vi "createEventForceActuatorInfo.vi"(8 "error in (no error)":errorcluster, 11 "UserEvents in":refnum<class "UserEvents.lvclass">) -> (0 "error out":errorcluster, 3 "UserEvents out":refnum<class "UserEvents.lvclass">)   [LabVIEW 2016, in "UserEvents.lvclass"]
uses:
  UserEvents.lvclass
  DataTypes/Topics/EventForceActuatorInfo.ctl
  DataTypes/Topics/Parts/Timestamp.ctl
  UserEvents.lvclass/UserEvents.ctl
  DataTypes/Topics/M1M3SupportTopics.lvlib
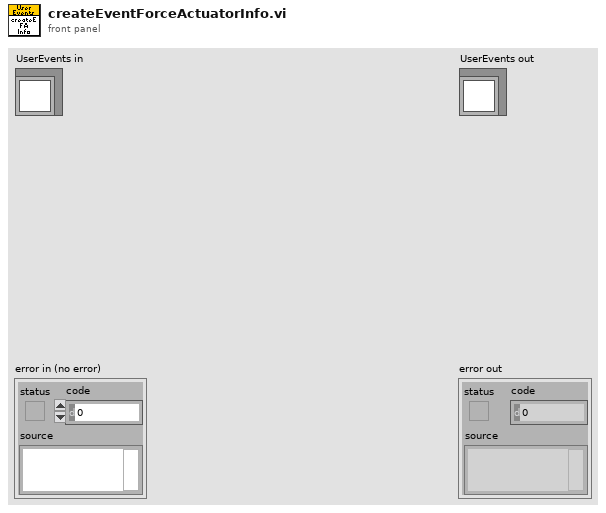
[diagram p1: front panel]
types:
  T1 = typedef "M1M3SupportTopics.lvlib/EventForceActuatorInfo.ctl" = cluster{"Timestamp":T2, "ReferenceId":i32[], "XPosition":sgl[], "YPosition":sgl[], "ZPosition":sgl[], "ILCUniqueId":i64[], "ILCApplicationType":u8[], "NetworkNodeType":u8[], "ILCSelectedOptions":u8[], "NetworkNodeOptions":u8[], "MajorRevision":u8[], "MinorRevision":u8[], "ADCScanRate":u8[], "MainADCCalibrationK1":sgl[], "MainADCCalibrationK2":sgl[], "MainADCCalibrationK3":sgl[], "MainADCCalibrationK4":sgl[], "MainAxialLoadCellOffset":sgl[], "MainLateralLoadCellOffset":sgl[], "MainAxialLoadCellSensitivity":sgl[], "MainLateralLoadCellSensitivity":sgl[], "BackupADCCalibrationK1":sgl[], "BackupADCCalibrationK2":sgl[], "BackupADCCalibrationK3":sgl[], "BackupADCCalibrationK4":sgl[], "BackupAxialLoadCellOffset":sgl[], "BackupLateralLoadCellOffset":sgl[], "BackupAxialLoadCellSensitivity":sgl[], "BackupLateralLoadCellSensitivity":sgl[], "DCAAxialGain":sgl[], "DCALateralGain":sgl[], "DCAUniqueId":i64[], "DCAFirmwareType":u8[], "DCAMajorRevision":u8[], "DCAMinorRevision":u8[], "MainCalibrationError":bool[], "BackupCalibrationError":bool[], "DCAFirmwareUpdate":bool[], "UniqueIdCRCError":bool[], "ApplicationTypeMismatch":bool[], "ApplicationMissing":bool[], "ApplicationCRCMismatch":bool[], "OneWireMissing":bool[], "OneWire1Mismatch":bool[], "OneWire2Mismatch":bool[], "DCAUniqueIdCRCError":bool[], "DCAMainCalibrationError":bool[], "DCABackupCalibrationError":bool[], "DCAApplicationMissing":bool[], "DCAApplicationCRCMismatch":bool[], "DCABootloaderActive":bool[]}
  T2 = typedef "M1M3SupportTopics.lvlib/Timestamp.ctl" = dbl
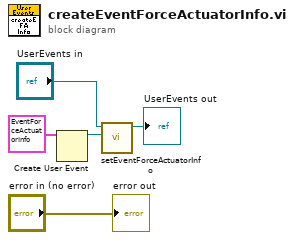
[diagram p0: block diagram]
diagram:
  n1 = Create User Event(user event datatype=T1 {"Timestamp"=0.0, "ReferenceId"=[], "XPosition"=[], "YPosition"=[], "ZPosition"=[], "ILCUniqueId"=[], "ILCApplicationType"=[], "NetworkNodeType"=[], "ILCSelectedOptions"=[], "NetworkNodeOptions"=[], "MajorRevision"=[], "MinorRevision"=[], "ADCScanRate"=[], "MainADCCalibrationK1"=[], "MainADCCalibrationK2"=[], "MainADCCalibrationK3"=[], "MainADCCalibrationK4"=[], "MainAxialLoadCellOffset"=[], "MainLateralLoadCellOffset"=[], "MainAxialLoadCellSensitivity"=[], "MainLateralLoadCellSensitivity"=[], "BackupADCCalibrationK1"=[], "BackupADCCalibrationK2"=[], "BackupADCCalibrationK3"=[], "BackupADCCalibrationK4"=[], "BackupAxialLoadCellOffset"=[], "BackupLateralLoadCellOffset"=[], "BackupAxialLoadCellSensitivity"=[], "BackupLateralLoadCellSensitivity"=[], "DCAAxialGain"=[], "DCALateralGain"=[], "DCAUniqueId"=[], "DCAFirmwareType"=[], "DCAMajorRevision"=[], "DCAMinorRevision"=[], "MainCalibrationError"=[], "BackupCalibrationError"=[], "DCAFirmwareUpdate"=[], "UniqueIdCRCError"=[], "ApplicationTypeMismatch"=[], "ApplicationMissing"=[], "ApplicationCRCMismatch"=[], "OneWireMissing"=[], "OneWire1Mismatch"=[], "OneWire2Mismatch"=[], "DCAUniqueIdCRCError"=[], "DCAMainCalibrationError"=[], "DCABackupCalibrationError"=[], "DCAApplicationMissing"=[], "DCAApplicationCRCMismatch"=[], "DCABootloaderActive"=[]} ("EventForceActuatorInfo")) -> (user event=w3:refnum<user-event>)  [unwired: 1 in, 1 out]
  n2 = call "setEventForceActuatorInfo.vi"("EventForceActuatorInfo"=w3, "UserEvents in"="UserEvents in") -> ("UserEvents out"=→"UserEvents out":refnum<class "UserEvents.lvclass">)  [unwired: 9 in]
  "error out" <- "error in (no error)"
